vi "Cycling_No_DAQ_Tasks_RT - 2C.vi"() -> ()   [LabVIEW 2020]
panel:
  out "PS Visa Out 3":refnum<visa-resource-name>
  out "PS error out 3":errorcluster
  in  "PS error in 3":errorcluster caption="PS error in (no error)"
  out "PS Visa Out 2":refnum<visa-resource-name>
  out "PS error out 2":errorcluster
  in  "PS error in 2":errorcluster caption="PS error in (no error)"
  out "PS error out":errorcluster
  out "PS Visa Out":refnum<visa-resource-name>
  in  "PS error in":errorcluster caption="PS error in (no error)"
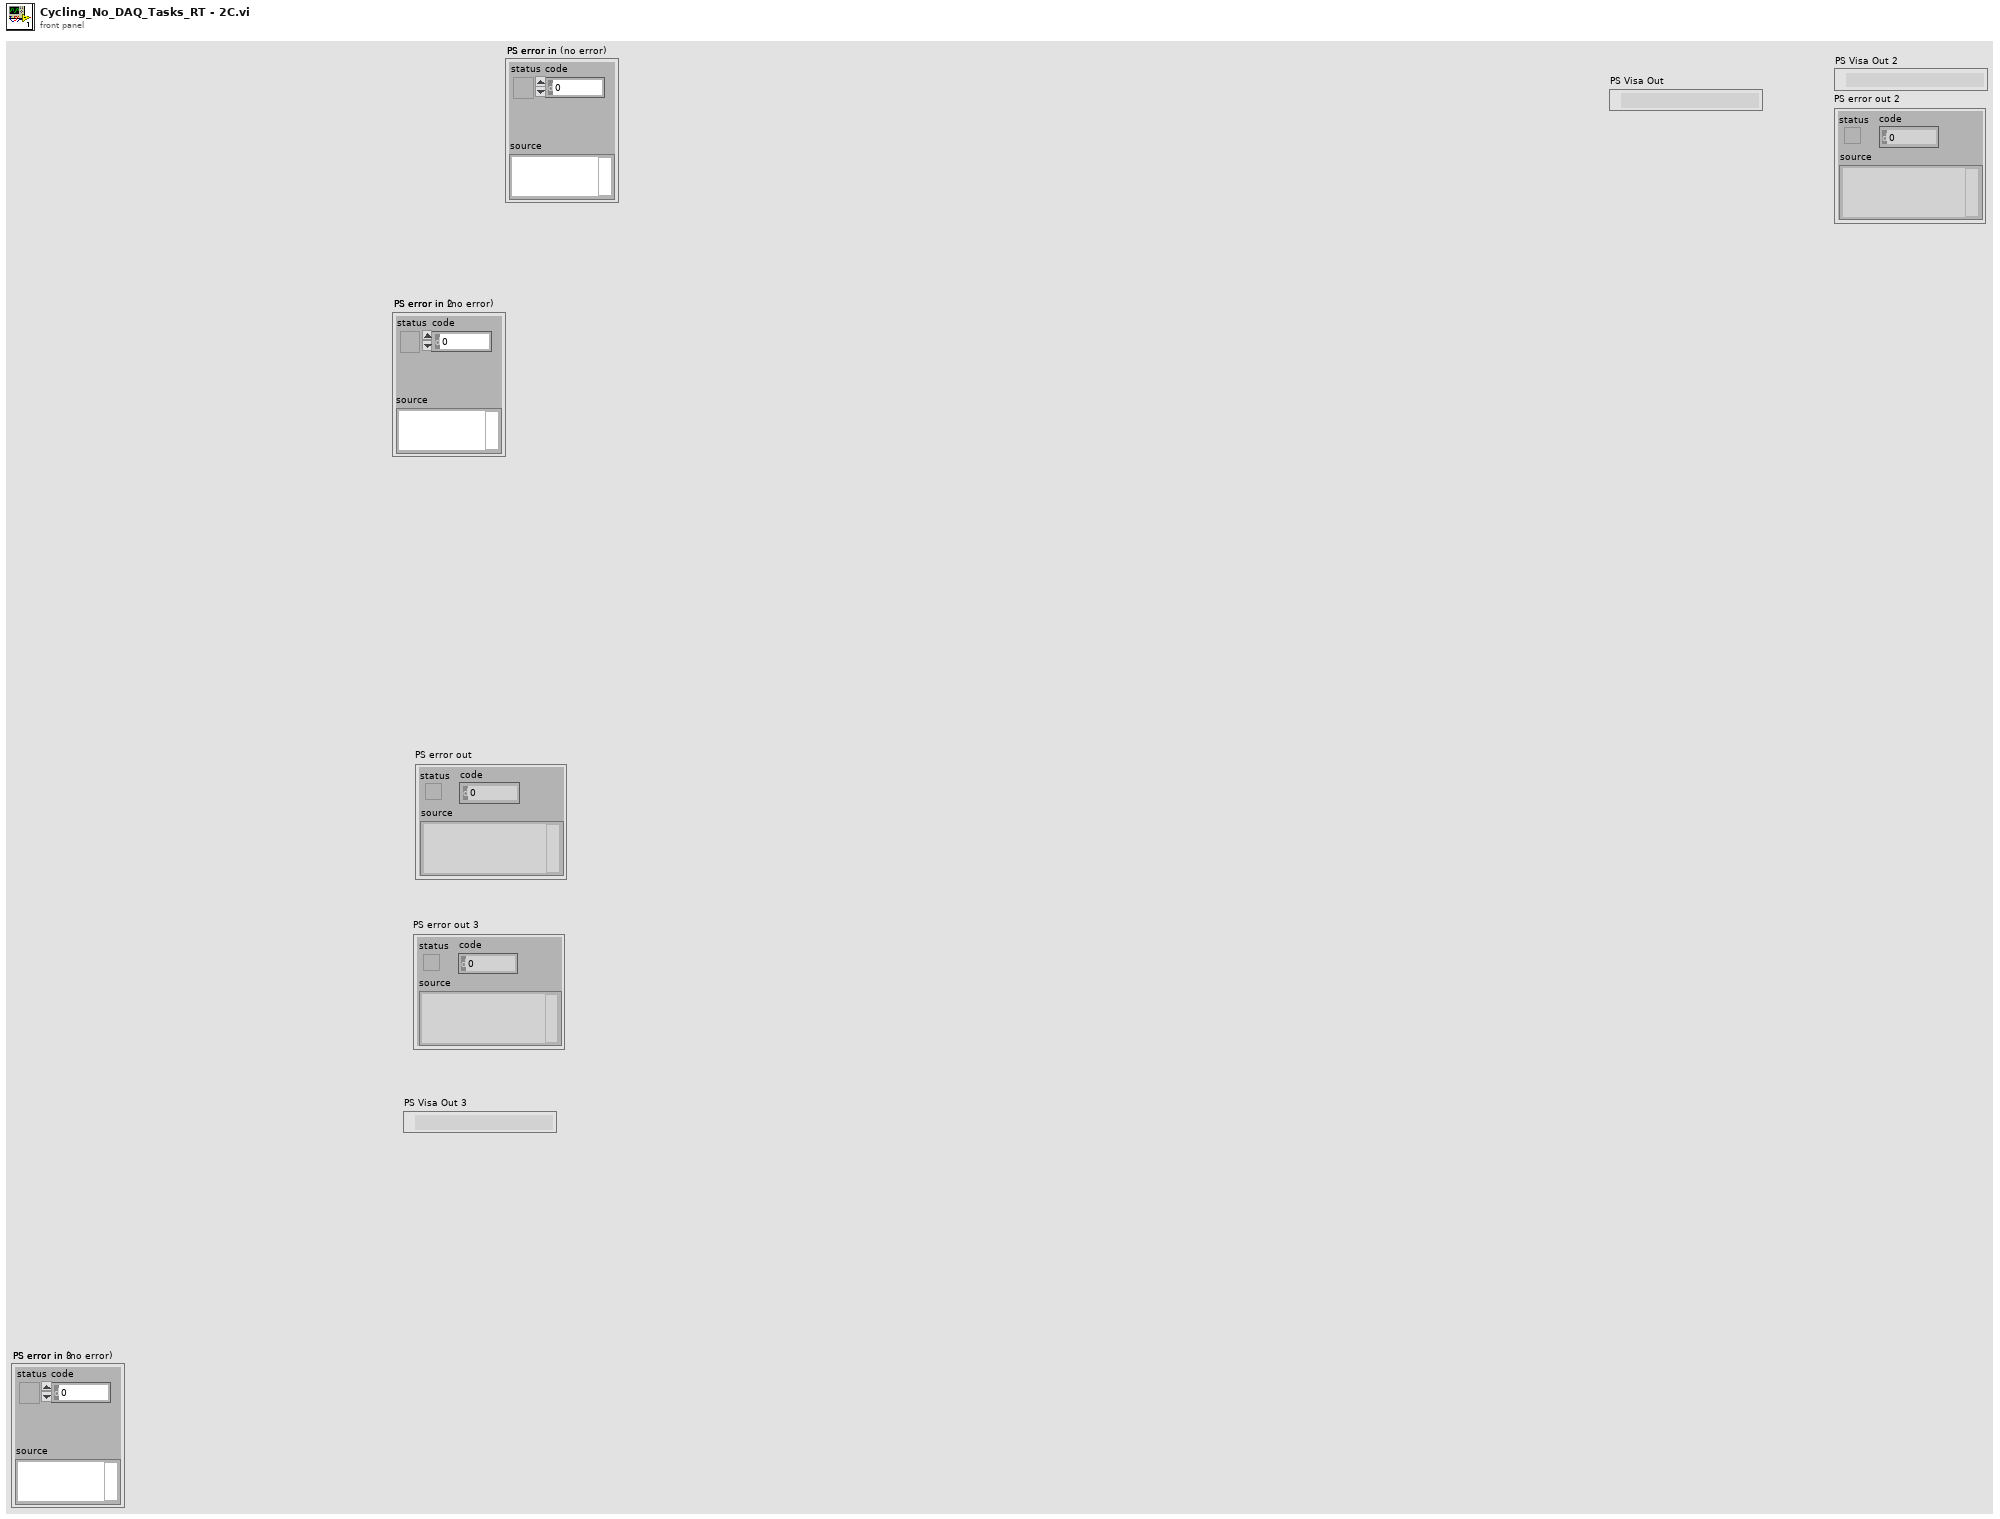
[diagram p1: front panel]
types:
  T1 = enum16{"\"30Q\"", "\"40T\"", "\"2P30Q\"", "\"3P30Q\"", "\"Nissan Leaf\""}
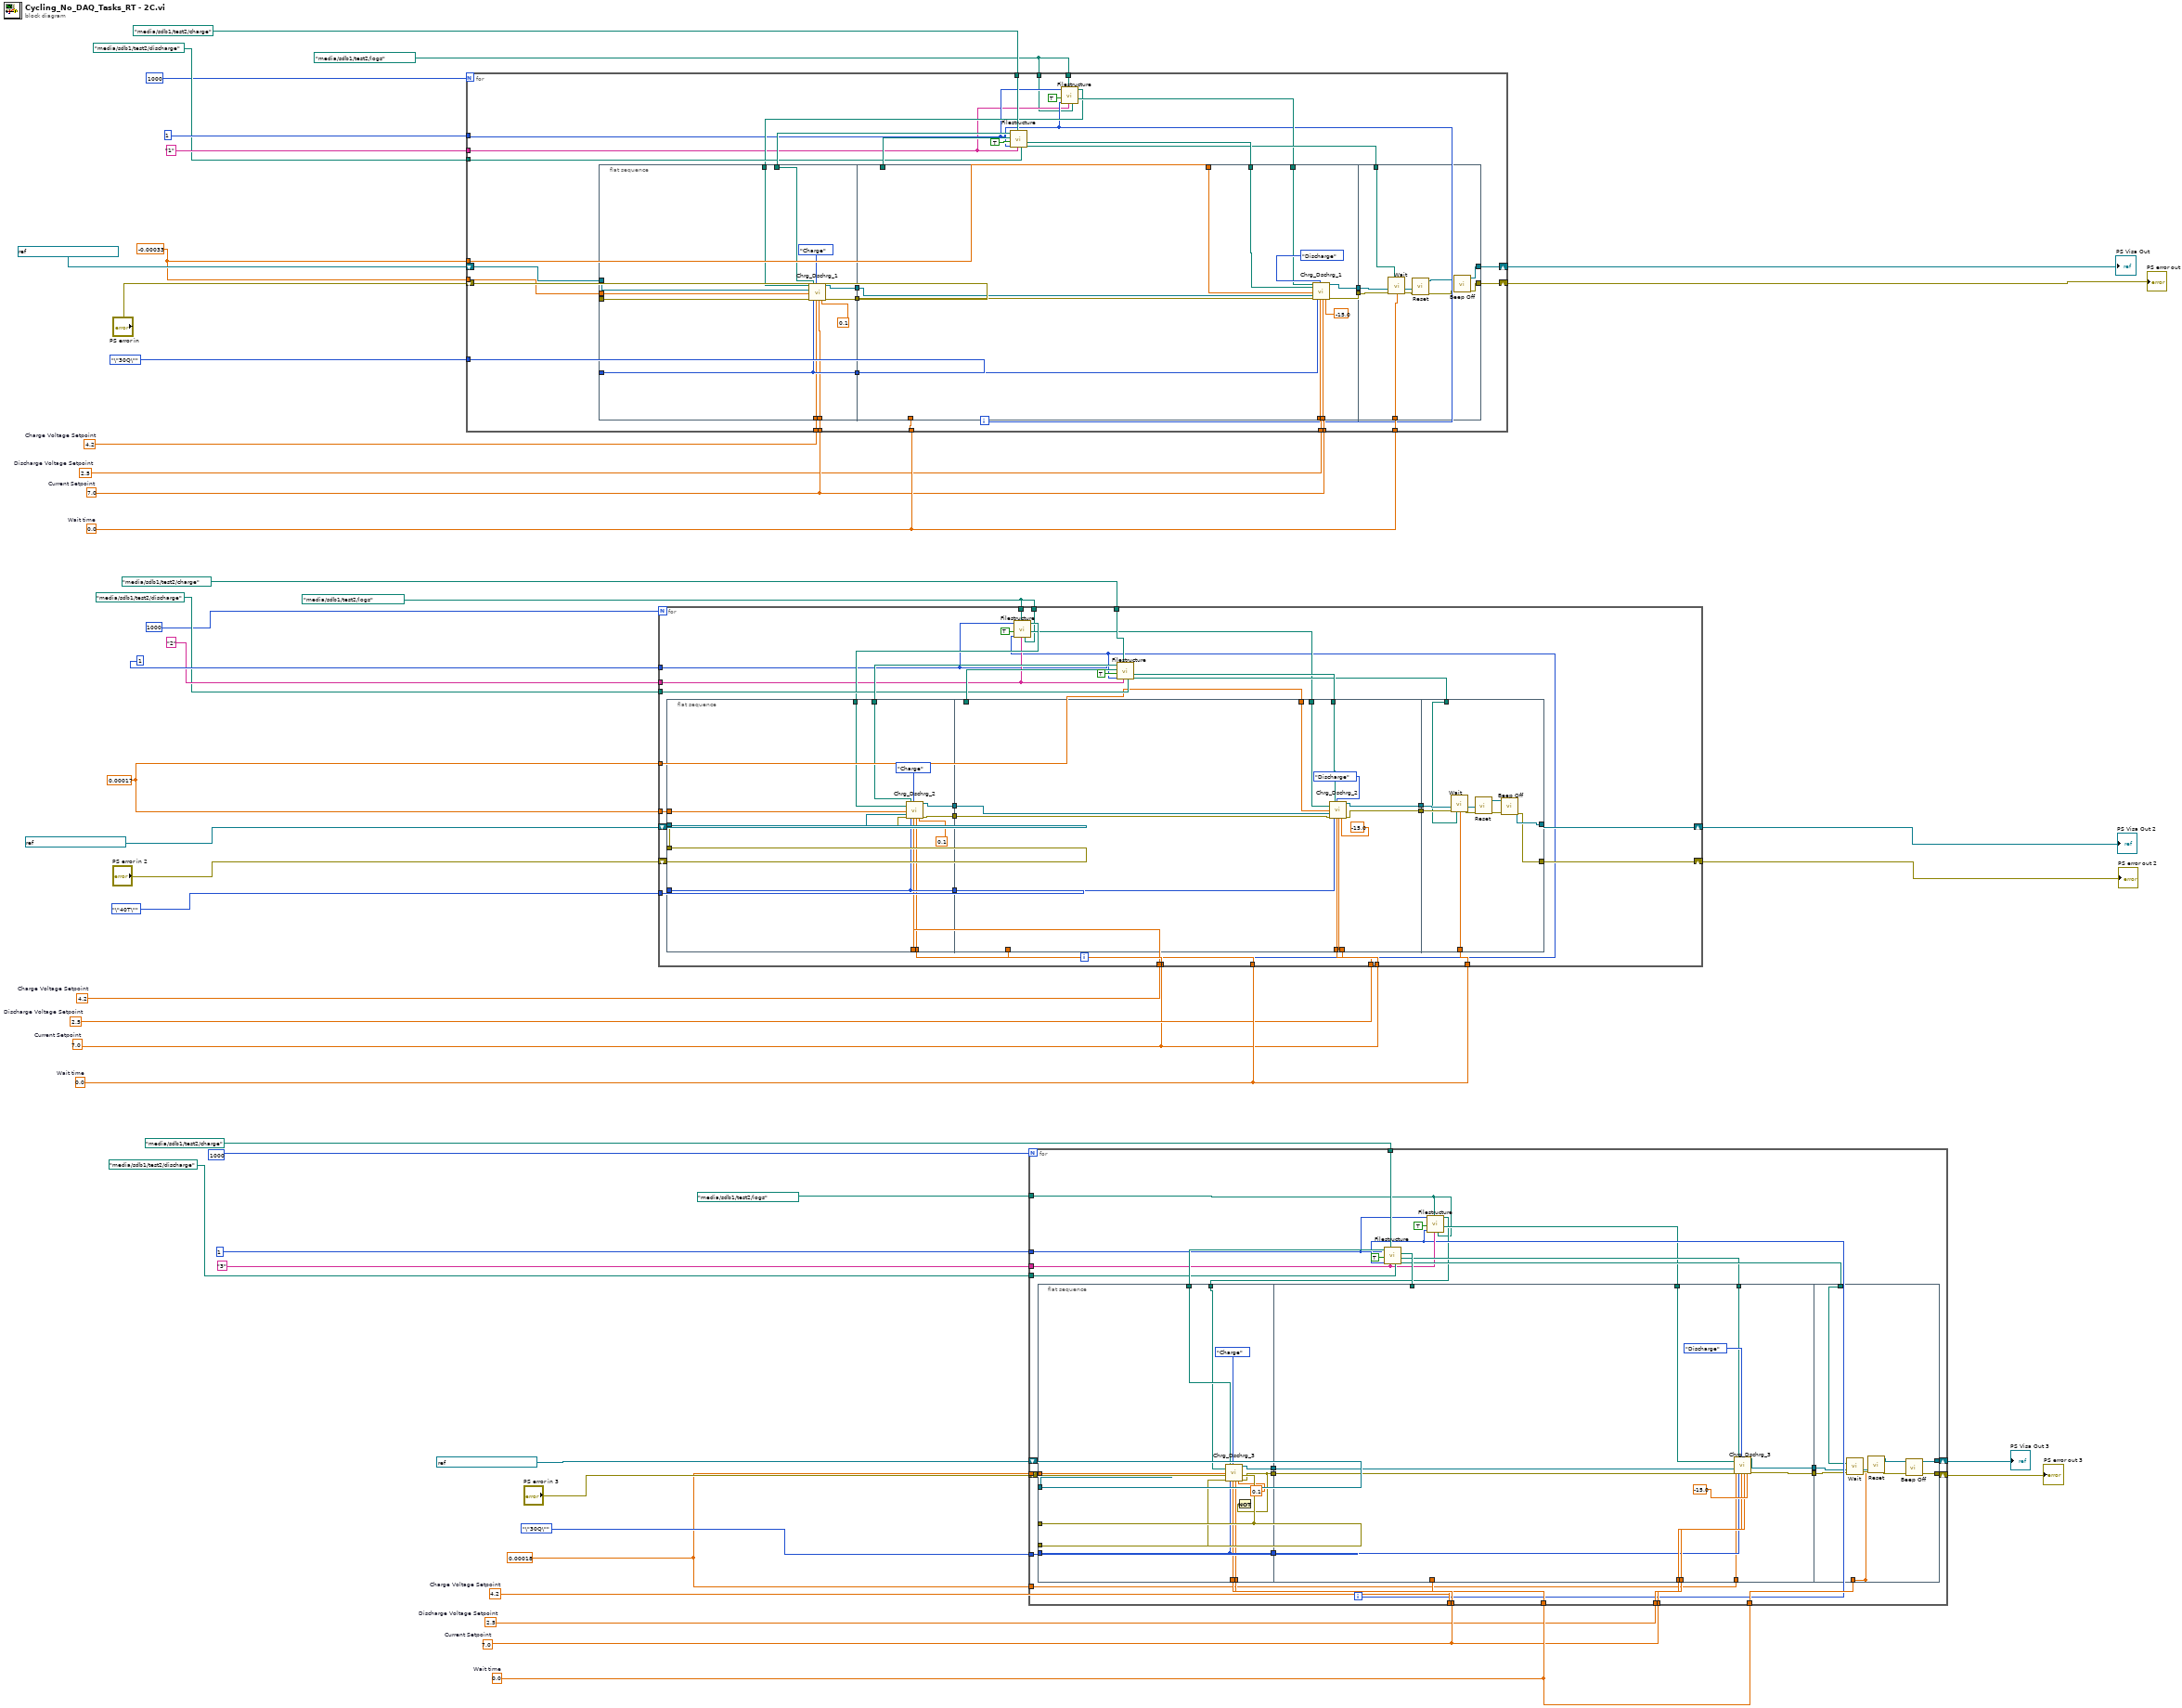
[diagram p0: block diagram]
diagram:
  w2 = path "/media/sdb1/test2/logs" ("Error log filepath")
  w3 = path "/media/sdb1/test2/logs" ("Error log filepath")
  w4 = 0.00018 ("Strain Offset")
  w5 = 0.00017 ("Strain Offset")
  w6 = 2.5  # Discharge Voltage Setpoint
  w9 = 0.0  # Wait time
  w7 = 7.0  # Current Setpoint
  w8 = 4.2  # Charge Voltage Setpoint
  w12 = 2.5  # Discharge Voltage Setpoint
  w13 = 0.0  # Wait time
  w11 = 7.0  # Current Setpoint
  w10 = 4.2  # Charge Voltage Setpoint
  w14 = 2.5  # Discharge Voltage Setpoint
  w17 = -0.00033 ("Strain Offset")
  w18 = 0.0  # Wait time
  w16 = 7.0  # Current Setpoint
  w15 = 4.2  # Charge Voltage Setpoint
  n1 = for {
    N: 1000 ("Number of Cycles") -> [_]
    tunnel: T1."\"30Q\"" ("Battery Type") -> [w74]
    tunnel: w15 -> [w73]
    tunnel: w16 -> [w72]
    tunnel: w18 -> [w63]
    shift-right: [w58] -> w45
    shift-left: refnum<visa-resource-name> "TCPIP0::192.168.0.246::inst0::INSTR" ("PS VISA in") -> [w76]
    shift-right: [w57] -> w46
    shift-left: "PS error in" -> [w75]
    tunnel: 1 ("Starting Cycle") -> [w51]
    tunnel: "1" ("Batteryname") -> [w50]
    tunnel: path "/media/sdb1/test2/discharge" ("Discharge filepath") -> [w66]
    tunnel: path "/media/sdb1/test2/charge" ("Charge filepath") -> [w65]
    tunnel: w18 -> [w64]
    tunnel: w17 -> [w62]
    tunnel: w17 -> [w61]
    tunnel: w16 -> [w60]
    tunnel: w14 -> [w59]
    tunnel: w2 -> [w55]
    tunnel: w2 -> [w49]
    i -> [w52]
    n2 = flat-sequence {
      tunnel: w76 -> [w87]
      tunnel: w75 -> [w88]
      tunnel: w74 -> [w89]
      tunnel: w73 -> [w84]
      tunnel: [w91] -> w81
      tunnel: [w83] -> w80
      tunnel: [w89] -> w79
      tunnel: w71 -> [w92]
      tunnel: w62 -> [w86]
      tunnel: w60 -> [w85]
      tunnel: w53 -> [w82]
      tunnel: w59 -> [w103]
      tunnel: w72 -> [w104]
      tunnel: w69 -> [w101]
      tunnel: [w99] -> w78
      tunnel: [w98] -> w77
      tunnel: w61 -> [w97]
      tunnel: w54 -> [w96]
      tunnel: w63 -> [_]
      tunnel: w70 -> [_]
      tunnel: w79 -> [w102]
      tunnel: w80 -> [w94]
      tunnel: w81 -> [w95]
      tunnel: w68 -> [w110]
      tunnel: w78 -> [w115]
      tunnel: w77 -> [w114]
      tunnel: w64 -> [w111]
      tunnel: [w107] -> w58
      tunnel: [w106] -> w57
      frame #0 {
        n3 = call "Chrg_Dschrg_1.vi"("Error log filepath"=w82, "Strain Offset"=w86, "PS VISA in"=w87, "PS error in"=w88, "CyclePath"=w92, "Battery Type"=w89, "Charge/discharge"=enum8{"Charge", "Discharge"}."Charge", "Charge/Discharge Voltage Setpoint"=w84, "Current Setpoint"=w85, "Current Cutoff"=0.1) -> ("PS VISA out"=w91:refnum<visa-resource-name>, "PS error out"=w83:errorcluster)  [unwired: 8 in]
      }
      frame #1 {
        n4 = call "Chrg_Dschrg_1.vi"("Error log filepath"=w96, "Strain Offset"=w97, "PS VISA in"=w95, "PS error in"=w94, "CyclePath"=w101, "Battery Type"=w102, "Charge/discharge"=enum8{"Charge", "Discharge"}."Discharge", "Charge/Discharge Voltage Setpoint"=w103, "Current Setpoint"=w104, "Current Cutoff"=-15.0) -> ("PS VISA out"=w99:refnum<visa-resource-name>, "PS error out"=w98:errorcluster)  [unwired: 8 in]
      }
      frame #2 {
        n5 = call "Wait.vi"("PS VISA in"=w115, "PS error in"=w114, "Wait Filepath"=w110, "Wait time"=w111) -> ("PS Visa Out"=w113:refnum<visa-resource-name>, "PS error out"=w112:errorcluster)  [unwired: 10 in]
        n6 = call "Reset.vi"("error in"=w112, "VISA resource name"=w113) -> ("error out"=w108:errorcluster, "VISA resource name out"=w109:refnum<visa-resource-name>)  [unwired: 8 in]
        n7 = call "Beep Off.vi"("error in"=w108, "VISA resource name"=w109) -> ("error out"=w106:errorcluster, "VISA resource name out"=w107:refnum<visa-resource-name>)  [unwired: 8 in]
      }
    }
    n8 = call "Filestructure.vi"("Discharge filepath"=w66, "Batteryname"=w50, "Charge filepath"=w65, "For loop i"=w52, "In for loop"=TRUE, "Starting Cycle"=w51) -> ("DischargeWaitPath"=w68:path, "DischargeCyclePath"=w69:path, "ChargeWaitPath"=w70:path, "ChargeCyclePath"=w71:path)  [unwired: 1 in, 1 out]
    n9 = call "Filestructure.vi"("Discharge filepath"=w49, "Batteryname"=w50, "Charge filepath"=w55, "For loop i"=w52, "In for loop"=TRUE, "Starting Cycle"=w51) -> ("DischargeCyclePath"=w54:path, "ChargeCyclePath"=w53:path)  [unwired: 1 in, 3 out]
  }
  "PS error out" <- w46
  "PS Visa Out" <- w45
  n10 = for {
    N: 1000 ("Number of Cycles") -> [_]
    tunnel: T1."\"40T\"" ("Battery Type") -> [w141]
    tunnel: w11 -> [w140]
    tunnel: w11 -> [w139]
    shift-right: [w134] -> w35
    shift-left: refnum<visa-resource-name> "TCPIP0::192.168.0.247::inst0::INSTR" ("PS VISA in") -> [w143]
    shift-right: [w130] -> w36
    shift-left: "PS error in 2" -> [w142]
    tunnel: 1 ("Starting Cycle") -> [w119]
    tunnel: "2" ("Batteryname 2") -> [w120]
    tunnel: path "/media/sdb1/test2/discharge" ("Discharge filepath") -> [w132]
    tunnel: path "/media/sdb1/test2/charge" ("Charge filepath") -> [w131]
    tunnel: w13 -> [w129]
    tunnel: w13 -> [w128]
    tunnel: w12 -> [w127]
    tunnel: w10 -> [w126]
    tunnel: w5 -> [w125]
    tunnel: w5 -> [w124]
    tunnel: w3 -> [w117]
    tunnel: w3 -> [w116]
    i -> [w118]
    n11 = flat-sequence {
      tunnel: w143 -> [w154]
      tunnel: w142 -> [w155]
      tunnel: w141 -> [w156]
      tunnel: w140 -> [w157]
      tunnel: [w153] -> w148
      tunnel: [w150] -> w147
      tunnel: [w156] -> w146
      tunnel: w138 -> [w159]
      tunnel: w126 -> [w152]
      tunnel: w125 -> [w151]
      tunnel: w122 -> [w149]
      tunnel: w127 -> [w170]
      tunnel: w139 -> [w171]
      tunnel: w136 -> [w168]
      tunnel: [w166] -> w145
      tunnel: [w165] -> w144
      tunnel: w124 -> [w164]
      tunnel: w121 -> [w163]
      tunnel: w128 -> [_]
      tunnel: w137 -> [_]
      tunnel: w146 -> [w169]
      tunnel: w147 -> [w161]
      tunnel: w148 -> [w162]
      tunnel: w135 -> [w177]
      tunnel: w145 -> [w182]
      tunnel: w144 -> [w181]
      tunnel: w129 -> [w178]
      tunnel: [w176] -> w134
      tunnel: [w173] -> w130
      frame #0 {
        n12 = call "Chrg_Dschrg_2.vi"("Error log filepath"=w149, "Strain Offset"=w151, "PS VISA in"=w154, "PS error in"=w155, "CyclePath"=w159, "Battery Type"=w156, "Charge/discharge"=enum8{"Charge", "Discharge"}."Charge", "Charge/Discharge Voltage Setpoint"=w152, "Current Setpoint"=w157, "Current Cutoff"=0.1) -> ("PS VISA out"=w153:refnum<visa-resource-name>, "PS error out"=w150:errorcluster)  [unwired: 8 in]
      }
      frame #1 {
        n13 = call "Chrg_Dschrg_2.vi"("Error log filepath"=w163, "Strain Offset"=w164, "PS VISA in"=w162, "PS error in"=w161, "CyclePath"=w168, "Battery Type"=w169, "Charge/discharge"=enum8{"Charge", "Discharge"}."Discharge", "Charge/Discharge Voltage Setpoint"=w170, "Current Setpoint"=w171, "Current Cutoff"=-15.0) -> ("PS VISA out"=w166:refnum<visa-resource-name>, "PS error out"=w165:errorcluster)  [unwired: 8 in]
      }
      frame #2 {
        n14 = call "Wait.vi"("PS VISA in"=w182, "PS error in"=w181, "Wait Filepath"=w177, "Wait time"=w178) -> ("PS Visa Out"=w180:refnum<visa-resource-name>, "PS error out"=w179:errorcluster)  [unwired: 10 in]
        n15 = call "Reset.vi"("error in"=w179, "VISA resource name"=w180) -> ("error out"=w174:errorcluster, "VISA resource name out"=w175:refnum<visa-resource-name>)  [unwired: 8 in]
        n16 = call "Beep Off.vi"("error in"=w174, "VISA resource name"=w175) -> ("error out"=w173:errorcluster, "VISA resource name out"=w176:refnum<visa-resource-name>)  [unwired: 8 in]
      }
    }
    n17 = call "Filestructure.vi"("Discharge filepath"=w116, "Batteryname"=w120, "Charge filepath"=w117, "For loop i"=w118, "In for loop"=TRUE, "Starting Cycle"=w119) -> ("DischargeCyclePath"=w121:path, "ChargeCyclePath"=w122:path)  [unwired: 1 in, 3 out]
    n18 = call "Filestructure.vi"("Discharge filepath"=w132, "Batteryname"=w120, "Charge filepath"=w131, "For loop i"=w118, "In for loop"=TRUE, "Starting Cycle"=w119) -> ("DischargeWaitPath"=w135:path, "DischargeCyclePath"=w136:path, "ChargeWaitPath"=w137:path, "ChargeCyclePath"=w138:path)  [unwired: 1 in, 1 out]
  }
  "PS error out 2" <- w36
  "PS Visa Out 2" <- w35
  n19 = for {
    N: 1000 ("Number of Cycles") -> [_]
    tunnel: T1."\"30Q\"" ("Battery Type") -> [w208]
    tunnel: w7 -> [w207]
    tunnel: w7 -> [w206]
    tunnel: w9 -> [w202]
    shift-right: [w201] -> w25
    shift-left: refnum<visa-resource-name> "TCPIP0::192.168.0.248::inst0::INSTR" ("PS VISA in") -> [w209]
    shift-right: [w197] -> w26
    shift-left: "PS error in 3" -> [w192]
    tunnel: 1 ("Starting Cycle") -> [w186]
    tunnel: "3" ("Batteryname 3") -> [w188]
    tunnel: path "/media/sdb1/test2/discharge" ("Discharge filepath") -> [w199]
    tunnel: path "/media/sdb1/test2/charge" ("Charge filepath") -> [w198]
    tunnel: w9 -> [w196]
    tunnel: w8 -> [w195]
    tunnel: w6 -> [w194]
    tunnel: w4 -> [w193]
    tunnel: w4 -> [w191]
    tunnel: path "/media/sdb1/test2/logs" ("Error log filepath") -> [w183]
    i -> [w187]
    n20 = flat-sequence {
      tunnel: w209 -> [w219]
      tunnel: w192 -> [w220]
      tunnel: w208 -> [w221]
      tunnel: w207 -> [w222]
      tunnel: [w224] -> w214
      tunnel: [w216] -> w213
      tunnel: [w221] -> w212
      tunnel: w205 -> [w225]
      tunnel: w195 -> [w218]
      tunnel: w193 -> [w217]
      tunnel: w192 -> [_]
      tunnel: w184 -> [w215]
      tunnel: w194 -> [w236]
      tunnel: w206 -> [w237]
      tunnel: [w233] -> w211
      tunnel: [w232] -> w210
      tunnel: w191 -> [w231]
      tunnel: w190 -> [w230]
      tunnel: w185 -> [w229]
      tunnel: w202 -> [_]
      tunnel: w204 -> [_]
      tunnel: w212 -> [w235]
      tunnel: w213 -> [w228]
      tunnel: w214 -> [w227]
      tunnel: w203 -> [w244]
      tunnel: w211 -> [w248]
      tunnel: w210 -> [w247]
      tunnel: [w243] -> _
      tunnel: [w242] -> w201
      tunnel: [w239] -> w197
      tunnel: w196 -> [w243]
      frame #0 {
        n21 = call "Chrg_Dschrg_3.vi"("Error log filepath"=w215, "Strain Offset"=w217, "PS VISA in"=w219, "PS error in"=w220, "CyclePath"=w225, "Battery Type"=w221, "Charge/discharge"=enum8{"Charge", "Discharge"}."Charge", "Charge/Discharge Voltage Setpoint"=w218, "Current Setpoint"=w222, "Current Cutoff"=0.1) -> ("PS VISA out"=w224:refnum<visa-resource-name>, "PS error out"=w216:errorcluster)  [unwired: 8 in]
        n22 = Not(x=w216) -> ()  [unwired: 1 out]
      }
      frame #1 {
        n23 = call "Chrg_Dschrg_3.vi"("Error log filepath"=w229, "Strain Offset"=w231, "PS VISA in"=w227, "PS error in"=w228, "CyclePath"=w230, "Battery Type"=w235, "Charge/discharge"=enum8{"Charge", "Discharge"}."Discharge", "Charge/Discharge Voltage Setpoint"=w236, "Current Setpoint"=w237, "Current Cutoff"=-15.0) -> ("PS VISA out"=w233:refnum<visa-resource-name>, "PS error out"=w232:errorcluster)  [unwired: 8 in]
      }
      frame #2 {
        n24 = call "Wait.vi"("PS VISA in"=w248, "PS error in"=w247, "Wait Filepath"=w244, "Wait time"=w243) -> ("PS Visa Out"=w246:refnum<visa-resource-name>, "PS error out"=w245:errorcluster)  [unwired: 10 in]
        n25 = call "Reset.vi"("error in"=w245, "VISA resource name"=w246) -> ("error out"=w240:errorcluster, "VISA resource name out"=w241:refnum<visa-resource-name>)  [unwired: 8 in]
        n26 = call "Beep Off.vi"("error in"=w240, "VISA resource name"=w241) -> ("error out"=w239:errorcluster, "VISA resource name out"=w242:refnum<visa-resource-name>)  [unwired: 8 in]
      }
    }
    n27 = call "Filestructure.vi"("Discharge filepath"=w199, "Batteryname"=w188, "Charge filepath"=w198, "For loop i"=w187, "In for loop"=TRUE, "Starting Cycle"=w186) -> ("DischargeWaitPath"=w203:path, "DischargeCyclePath"=w190:path, "ChargeWaitPath"=w204:path, "ChargeCyclePath"=w205:path)  [unwired: 1 in, 1 out]
    n28 = call "Filestructure.vi"("Discharge filepath"=w183, "Batteryname"=w188, "Charge filepath"=w183, "For loop i"=w187, "In for loop"=TRUE, "Starting Cycle"=w186) -> ("DischargeCyclePath"=w185:path, "ChargeCyclePath"=w184:path)  [unwired: 1 in, 3 out]
  }
  "PS error out 3" <- w26
  "PS Visa Out 3" <- w25
